vi "Unit Test.vi"() -> ()   [LabVIEW 2019, in "IDEX.lvlib"]
uses:
  IDEX.lvlib
  User Event/Controls/UE Abort Action.ctl
panel:
  in  "VISA name":refnum<visa-resource-name>="visa://169.254.25.118/ASRL1::INSTR"
  out "Current Position":string
  in  "Initialize":bool
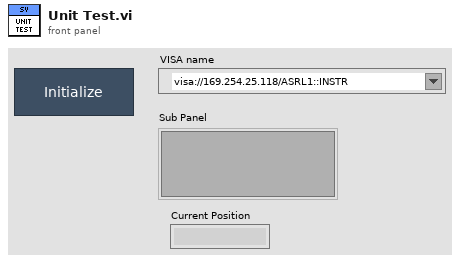
[diagram p1: front panel]
types:
  T1 = typedef "UE Abort Action.ctl" = enum16{"Create", "Get", "Destroy"}
  T2 = typedef "IDEX.lvlib/SEQ Data.ctl" = cluster{"Position":string, "Initialize Done?":bool, "VI Refnum":refnum<vi>}
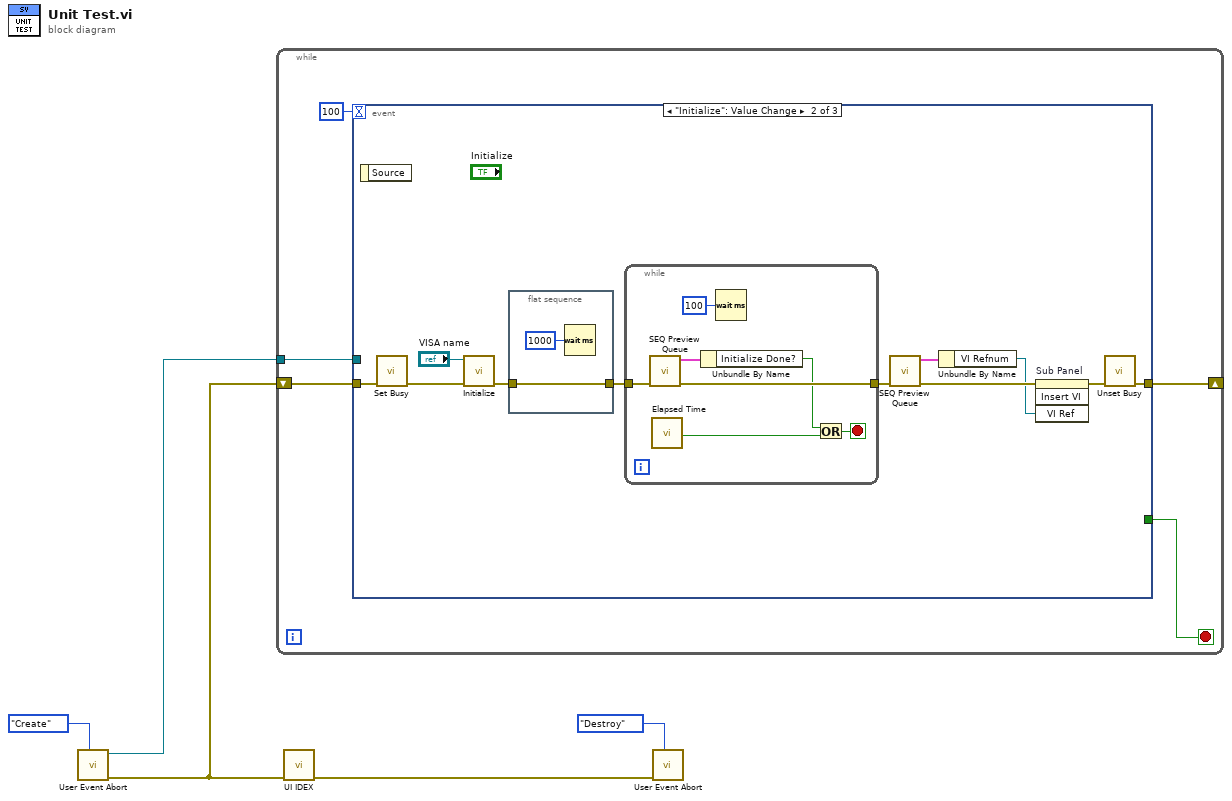
[diagram p0: block diagram]
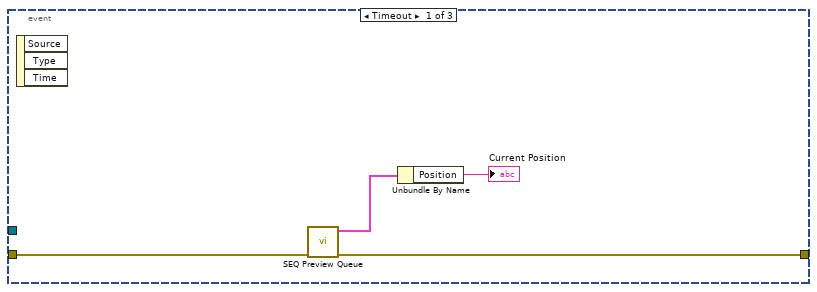
[diagram p2: hidden frame]
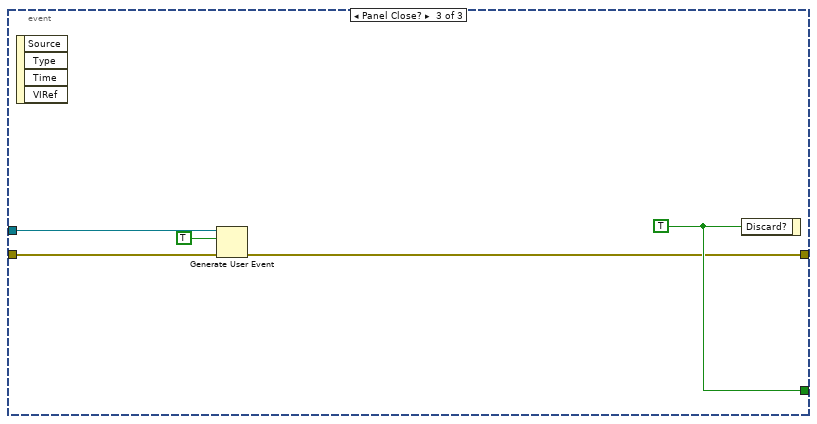
[diagram p3: hidden frame]
diagram:
  n1 = call "User Event Abort.vi"("Action"=UE_Abort_Action."Create") -> ("Error Out"=w1:errorcluster, "User Event Out"=w2:refnum<user-event>)  [unwired: 9 in]
  n2 = while {
    tunnel: w2 -> [w10]
    shift-right: [w7] -> _
    shift-left: w1 -> [w8]
    stop <- w9 stop-if-true
    n3 = event shown="[1] \"Initialize\": Value Change" {
      selector: _ -> [_ _ _]
      dyn-events: _ -> [_ _ _]
      timeout: 100 -> [_ _ _]
      tunnel: w10 -> [_ _ w38]
      tunnel: [_ _ w39] -> w9
      tunnel: w8 -> [w13 w25 w36]
      tunnel: [w12 w23 w35] -> w7
      event Timeout {
        n4 = event-data() -> ()  [unwired: 1 in, 3 out]
        n5 = call "SEQ Preview Queue.vi"("error in"=w13) -> ("error out"=w12:errorcluster, "SEQ Data"=w14:T2)  [unwired: 9 in]
        n6 = Unbundle By Name(w14) -> ("Position"=→"Current Position":string)
      }
      event "Initialize": Value Change {
        n7 = event-data() -> ()  [unwired: 1 in, 1 out]
        n8 = call <vilib>:"Set Busy.vi"("error in (no error)"=w25) -> ("error out"=w24:errorcluster)  [unwired: 9 in, 1 out]
        n9 = call "Initialize.vi"("Error In"=w24, "VISA name"="VISA name") -> ("Error Out"=w22:errorcluster)  [unwired: 9 in]
        n10 = flat-sequence {
          tunnel: w22 -> [w26]
          tunnel: [w26] -> w21
          frame #0 {
            n11 = Wait (ms)(milliseconds to wait=u32 1000) -> ()  [unwired: 1 out]
          }
        }
        n12 = while {
          tunnel: w21 -> [w33]
          tunnel: [w31] -> w20
          stop <- w28 stop-if-true
          n13 = call "SEQ Preview Queue.vi"("error in"=w33) -> ("error out"=w31:errorcluster, "SEQ Data"=w32:T2)  [unwired: 9 in]
          n14 = call "Elapsed Time"() -> ("Time has Elapsed"=w30:bool)  [unwired: 12 in, 7 out]
          n15 = Unbundle By Name(w32) -> ("Initialize Done?"=w29:bool)
          n16 = Wait (ms)(milliseconds to wait=u32 100) -> ()  [unwired: 1 out]
          n17 = Or(x=w29, y=w30) -> (x .or. y?=w28:bool)
        }
        n18 = call "SEQ Preview Queue.vi"("error in"=w20) -> ("error out"=w18:errorcluster, "SEQ Data"=w19:T2)  [unwired: 9 in]
        n19 = Unbundle By Name(w19) -> ("VI Refnum"=w16:refnum<vi>)
        n20 = invoke on="Sub Panel" class="SubPnl" method="Insert VI"(error in=w18, "VI Ref"=w16) -> (error out=w17:errorcluster)  [unwired: 2 in, 3 out]
        n21 = call <vilib>:"Unset Busy.vi"("error in (no error)"=w17) -> ("error out"=w23:errorcluster)  [unwired: 10 in]
      }
      event Panel Close? {
        w39 = TRUE ("Discard?")
        n22 = event-data() -> ()  [unwired: 1 in, 4 out]
        n23 = Generate User Event(user event=w38, event data cluster=TRUE ("event data"), error in=w36) -> (error out=w35:errorcluster)  [unwired: 1 in, 1 out]
        n24 = event-data("Discard?"=w39) -> ()  [unwired: 1 in, 1 out]
      }
    }
  }
  n25 = call "UI IDEX.vi"("error in"=w1) -> ("error out"=w5:errorcluster)  [unwired: 10 in]
  n26 = call "User Event Abort.vi"("Action"=UE_Abort_Action."Destroy", "Error In"=w5) -> ()  [unwired: 8 in, 2 out]
